vi "Vision_Processing_R_R5.vi"(0 "Current State":T6(ring)=enum."Short Range", 1 "Image Dst":T5=refnum, 2 "Inpute Image":T5=refnum, 3 "Startup Flag":bool, 5 "Current ROI Descriptor":T11={"Global Rectangle"=[0, 0, 320, 240], "Contours"=[{"ID"=enum."External", "Type"=12, "Coordinates"=[0, 0, 320, 240, 0]}]} {"Contours"."Type" items=["No Selection", "Point", "Line", "Rectangle", "Oval", "Polygon", "Freehand Region", "Annulus", "Unused2", "Unused3", "Broken Line", "Freehand Line", "Rotated Rectangle"]}, 6 "Avg Score - Last":dbl=802.5034383138021, 7 "error in (no error)":errorcluster, 8 "Current Settings":T9={"Curve Parameters"={"Extraction Mode"=1, "Edge Threshold"=150, "Edge Filter Size"=0, "Min Length"=25, "Row Search Step Size"=15, "Col Search Step Size"=15, "Max Endpoint Gap"=2, "Closed"=TRUE, "Subpixel"=TRUE}, "Match Mode"={"Rotation"=TRUE, "Scale"=TRUE, "Occlusion"=TRUE, "Reserved"=FALSE, "Reserved"=FALSE, "Reserved"=FALSE}, "Range Settings"=[{"Match Constraints"=0, "Min"=-5.0, "Max"=5.0}, {"Match Constraints"=1, "Min"=20.0, "Max"=150.0}, {"Match Constraints"=2, "Min"=0.0, "Max"=25.0}], "Number of Matches"=1, "Minimum Match Score"=800.0, "SubPixel Accuracy"=TRUE, "Adv. Geometric Match Options 2"=[{"Setup Data Item"=20, "Item Value"=0.0}, {"Setup Data Item"=22, "Item Value"=1.0}]} {"Curve Parameters"."Extraction Mode" items=["Normal", "Uniform Regions"]; "Curve Parameters"."Edge Filter Size" items=["Fine", "Normal", "Contour Tracing"]; "Curve Parameters"."Max Endpoint Gap" min=0; "Curve Parameters"."Col Search Step Size" min=1 max=255 step=1; "Curve Parameters"."Row Search Step Size" min=1 max=255 step=1; "Curve Parameters"."Min Length" min=0; "Curve Parameters"."Edge Threshold" min=1 max=350 step=1; "Range Settings"."Max" format="%.2f"; "Range Settings"."Min" format="%.2f"; "Range Settings"."Match Constraints" items=["Rotation Angle (degrees)", "Scale Factor (%)", "Occlusion (%)"]; "Adv. Geometric Match Options 2"."Setup Data Item" items=["Curve Extraction Mode", "Curve Edge Threshold", "Curve Edge Filter Size", "Min Curve Length", "Curve Row Search Step Size", "Curve Col Search Step Size", "Curve Max Endpoint Gap", "Extract Closed Curves", "Enable Subpixel Curve Extraction", "Enable Correlation Score", "Enable Subpixel Accuracy", "Subpixel Iterations", "Subpixel Tolerance", "Initial Match List Length", "Enable Target Template Curve Score", "Min Match Separation Distance", "Min Match Separation Angle", "Min Match Separation Scale", "Max Match Overlap", "Enable Coarse Result", "Enable Calibration Support", "Enable Contrast Reversal", "Search Strategy", "Refinement Match Factor", "Subpixel Match Factor"]}, 9 "Sub Beacon Search Enable":bool[](array[boolean])=[FALSE, FALSE, FALSE, FALSE, FALSE], 10 "History Data - IN":T4={"Valid Beacon History - in"=[FALSE, FALSE, FALSE, FALSE, FALSE, FALSE, FALSE, FALSE, FALSE, FALSE, FALSE, FALSE, FALSE, FALSE, FALSE, FALSE, FALSE, FALSE, FALSE, FALSE], "Valid Score History"=[916.1194458007812, 0.0, 921.171142578125, 952.2998657226562, 947.6416015625, 946.7607421875, 946.6710815429688, 913.2891235351562, 946.3783569335938, 946.1008911132812, 949.7362060546875, 948.7965087890625, 947.1905517578125, 948.5363159179688, 949.03466796875, 951.10986328125, 800.9814453125, 952.3334350585938, 926.0540161132812, 946.85888671875], "Valid Scale History"=[77.35153198242188, 0.0, 77.18988037109375, 76.20046997070312, 76.42532348632812, 76.47498321533203, 76.45317840576172, 77.11006927490234, 76.4490966796875, 76.39661407470703, 76.34481048583984, 76.36200714111328, 76.56851196289062, 76.3750228881836, 76.43797302246094, 76.20098876953125, 68.23258972167969, 76.18832397460938, 77.75858306884766, 76.44164276123047]} {"Valid Scale History" format="%#_13g"; "Valid Score History" format="%#_13g"}, 13 "Avg Scale - Last":dbl=73.9835688273112, 16 "History Size":i32=20) -> (11 "Avg Scale":dbl=73.9835688273112, 12 "Avg Score":dbl=802.5034383138021, 14 "Tracking Info":T1, 15 "Next Main ROI Descriptor":T2 {"Contours"."Type" items=["No Selection", "Point", "Line", "Rectangle", "Oval", "Polygon", "Freehand Region", "Annulus", "Unused2", "Unused3", "Broken Line", "Freehand Line", "Rotated Rectangle"]}, 17 "Beacon - Scales":sgl[](array[numeric])=[0.0, 0.0, 133.74268, 128.61499, 0.0], 18 "History Data - Out":T3={"Valid Beacon History\nOut"=[FALSE, FALSE, FALSE, FALSE, FALSE, FALSE, FALSE, FALSE, FALSE, FALSE, FALSE, FALSE, FALSE, FALSE, FALSE, FALSE, FALSE, FALSE, FALSE, FALSE], "Valid Score History\nOut"=[916.1194458007812, 0.0, 921.171142578125, 952.2998657226562, 947.6416015625, 946.7607421875, 946.6710815429688, 913.2891235351562, 946.3783569335938, 946.1008911132812, 949.7362060546875, 948.7965087890625, 947.1905517578125, 948.5363159179688, 949.03466796875, 951.10986328125, 800.9814453125, 952.3334350585938, 926.0540161132812, 946.85888671875], "Valid Scale History\nOut"=[77.35153198242188, 0.0, 77.18988037109375, 76.20046997070312, 76.42532348632812, 76.47498321533203, 76.45317840576172, 77.11006927490234, 76.4490966796875, 76.39661407470703, 76.34481048583984, 76.36200714111328, 76.56851196289062, 76.3750228881836, 76.43797302246094, 76.20098876953125, 68.23258972167969, 76.18832397460938, 77.75858306884766, 76.44164276123047]} {"Valid Scale History\nOut" format="%#_13g"; "Valid Score History\nOut" format="%#_13g"}, 19 "Y Coordinates":sgl[](array[numeric])=[0.0, 0.0, 133.74268, 128.61499, 0.0], 20 "Beacons Found":bool[](array[boolean])=[FALSE, FALSE, TRUE, TRUE, FALSE], 21 "X Coordinates":sgl[](array[numeric])=[0.0, 0.0, 162.26208, 213.98871, 0.0], 23 "Lock Status":bool, 24 "Startup Flag - out":bool, 25 "New Settings":T9={"Curve Parameters"={"Extraction Mode"=1, "Edge Threshold"=150, "Edge Filter Size"=0, "Min Length"=25, "Row Search Step Size"=15, "Col Search Step Size"=15, "Max Endpoint Gap"=2, "Closed"=TRUE, "Subpixel"=TRUE}, "Match Mode"={"Rotation"=TRUE, "Scale"=TRUE, "Occlusion"=TRUE, "Reserved"=FALSE, "Reserved"=FALSE, "Reserved"=FALSE}, "Range Settings"=[{"Match Constraints"=0, "Min"=-5.0, "Max"=5.0}, {"Match Constraints"=1, "Min"=20.0, "Max"=150.0}, {"Match Constraints"=2, "Min"=0.0, "Max"=25.0}], "Number of Matches"=1, "Minimum Match Score"=800.0, "SubPixel Accuracy"=TRUE, "Adv. Geometric Match Options 2"=[{"Setup Data Item"=20, "Item Value"=0.0}, {"Setup Data Item"=22, "Item Value"=1.0}]} {"Curve Parameters"."Extraction Mode" items=["Normal", "Uniform Regions"]; "Curve Parameters"."Edge Filter Size" items=["Fine", "Normal", "Contour Tracing"]; "Curve Parameters"."Max Endpoint Gap" min=0; "Curve Parameters"."Col Search Step Size" min=1 max=255 step=1; "Curve Parameters"."Row Search Step Size" min=1 max=255 step=1; "Curve Parameters"."Min Length" min=0; "Curve Parameters"."Edge Threshold" min=1 max=350 step=1; "Range Settings"."Max" format="%.2f"; "Range Settings"."Min" format="%.2f"; "Range Settings"."Match Constraints" items=["Rotation Angle (degrees)", "Scale Factor (%)", "Occlusion (%)"]}, 26 "Next State":T6(ring)=enum."Short Range", 27 "Right Image 2":T5(plugin-control))   [LabVIEW 2015]
uses:
  <vilib>/vision/Image Controls.llb/IMAQ Image.ctl
  <vilib>/vision/Pattern Matching.llb/IMAQ Curve Parameters.ctl
  <vilib>/vision/Pattern Matching.llb/IMAQ Match Range Setting.ctl
panel:
  in  "dimension size":i32=40
  in  "Divider (Filters 1)":sgl=1.0
  in  "SR / SCR\nTransition Scale":sgl=100.0
  in  "Score\nCushion- tight":dbl=75.0
  in  "Main ROI Decay\nper Fail (Vertical)":i32=5
  in  "ROI_factor(Horiztonal) SCR":sgl=1.7
  in  "ROI_factor(vertical) SCR":sgl=1.5
  in  "Dumping Range Beacon Filepath**":path=path "/home/lvuser/natinst/bin/BeaconTemplates/SCR_RIGHT.png"
  in  "Scale Decay \nFactor":dbl=0.5
  in  "Scale Decay \nFactor":dbl=5.0
  in  "Valid Treshold\nfor Lock":i16=3
  in  "Horiztonall Beacon \nCushion (pixels)":sgl=25.0
  out "New Min Score":dbl=800.0
  out "New Low Scale":dbl=20.0
  out "New high Scale":dbl=150.0
  in  "Absolute\nMinimum Score":dbl=700.0
  in  "Absolute\nMaximum Scale":dbl=300.0
  in  "Absolute\nMinimum Scale":dbl=10.0
  in  "Default No Lock\nSetting Values":T10={"Min Scale"=20.0, "Max Scale"=170.0, "Min Score"=800.0}
  in  "Score\nCushion":dbl=125.0
  in  "Scale \nCushion":dbl=7.0
  in  "LR to SR\nTransition Scale":sgl=80.0
  in  "SR /  LR\nTransition Scale":sgl=80.0
  in  "Timeout \nThrehsold":i32=1000
  in  "Main ROI Decay\nper Fail (Horiztonal)":i32=25
  in  "ROI_factor(Horiztonal) LR":sgl=5.0
  in  "ROI_factor(vertical) LR":sgl=1.5
  in  "ROI_factor(vertical) SR":sgl=2.7
  in  "ROI_factor(Horiztonal) SR":sgl=2.0
  out "Current  Score":sgl=916.11945
  out "Current  Scale":sgl=77.35153
  in  "Fail Count - In":i32
  in  "Sub Beacon Template File Path - ARRAY":path[](array[path])=[path "/home/lvuser/natinst/bin/BeaconTemplates/Sub1.png", path "/home/lvuser/natinst/bin/BeaconTemplates/Sub2.png", path "/home/lvuser/natinst/bin/BeaconTemplates/Sub3.png", path "/home/lvuser/natinst/bin/BeaconTemplates/Sub4.png", path "/home/lvuser/natinst/bin/BeaconTemplates/Sub5.png"]
  in  "Short Range Template FIle Path":path=path "/home/lvuser/natinst/bin/BeaconTemplates/SR_Right.png"
  in  "Long Range Main\nBeacon File Path":path=path "/home/lvuser/natinst/bin/BeaconTemplates/LR_Main.png"
  # "INPUTS"
  # "FILE PATHS"
  # "CONFIG"
  # "OUTPUTS"
  # "************"
  # "Range"
  # "Range"
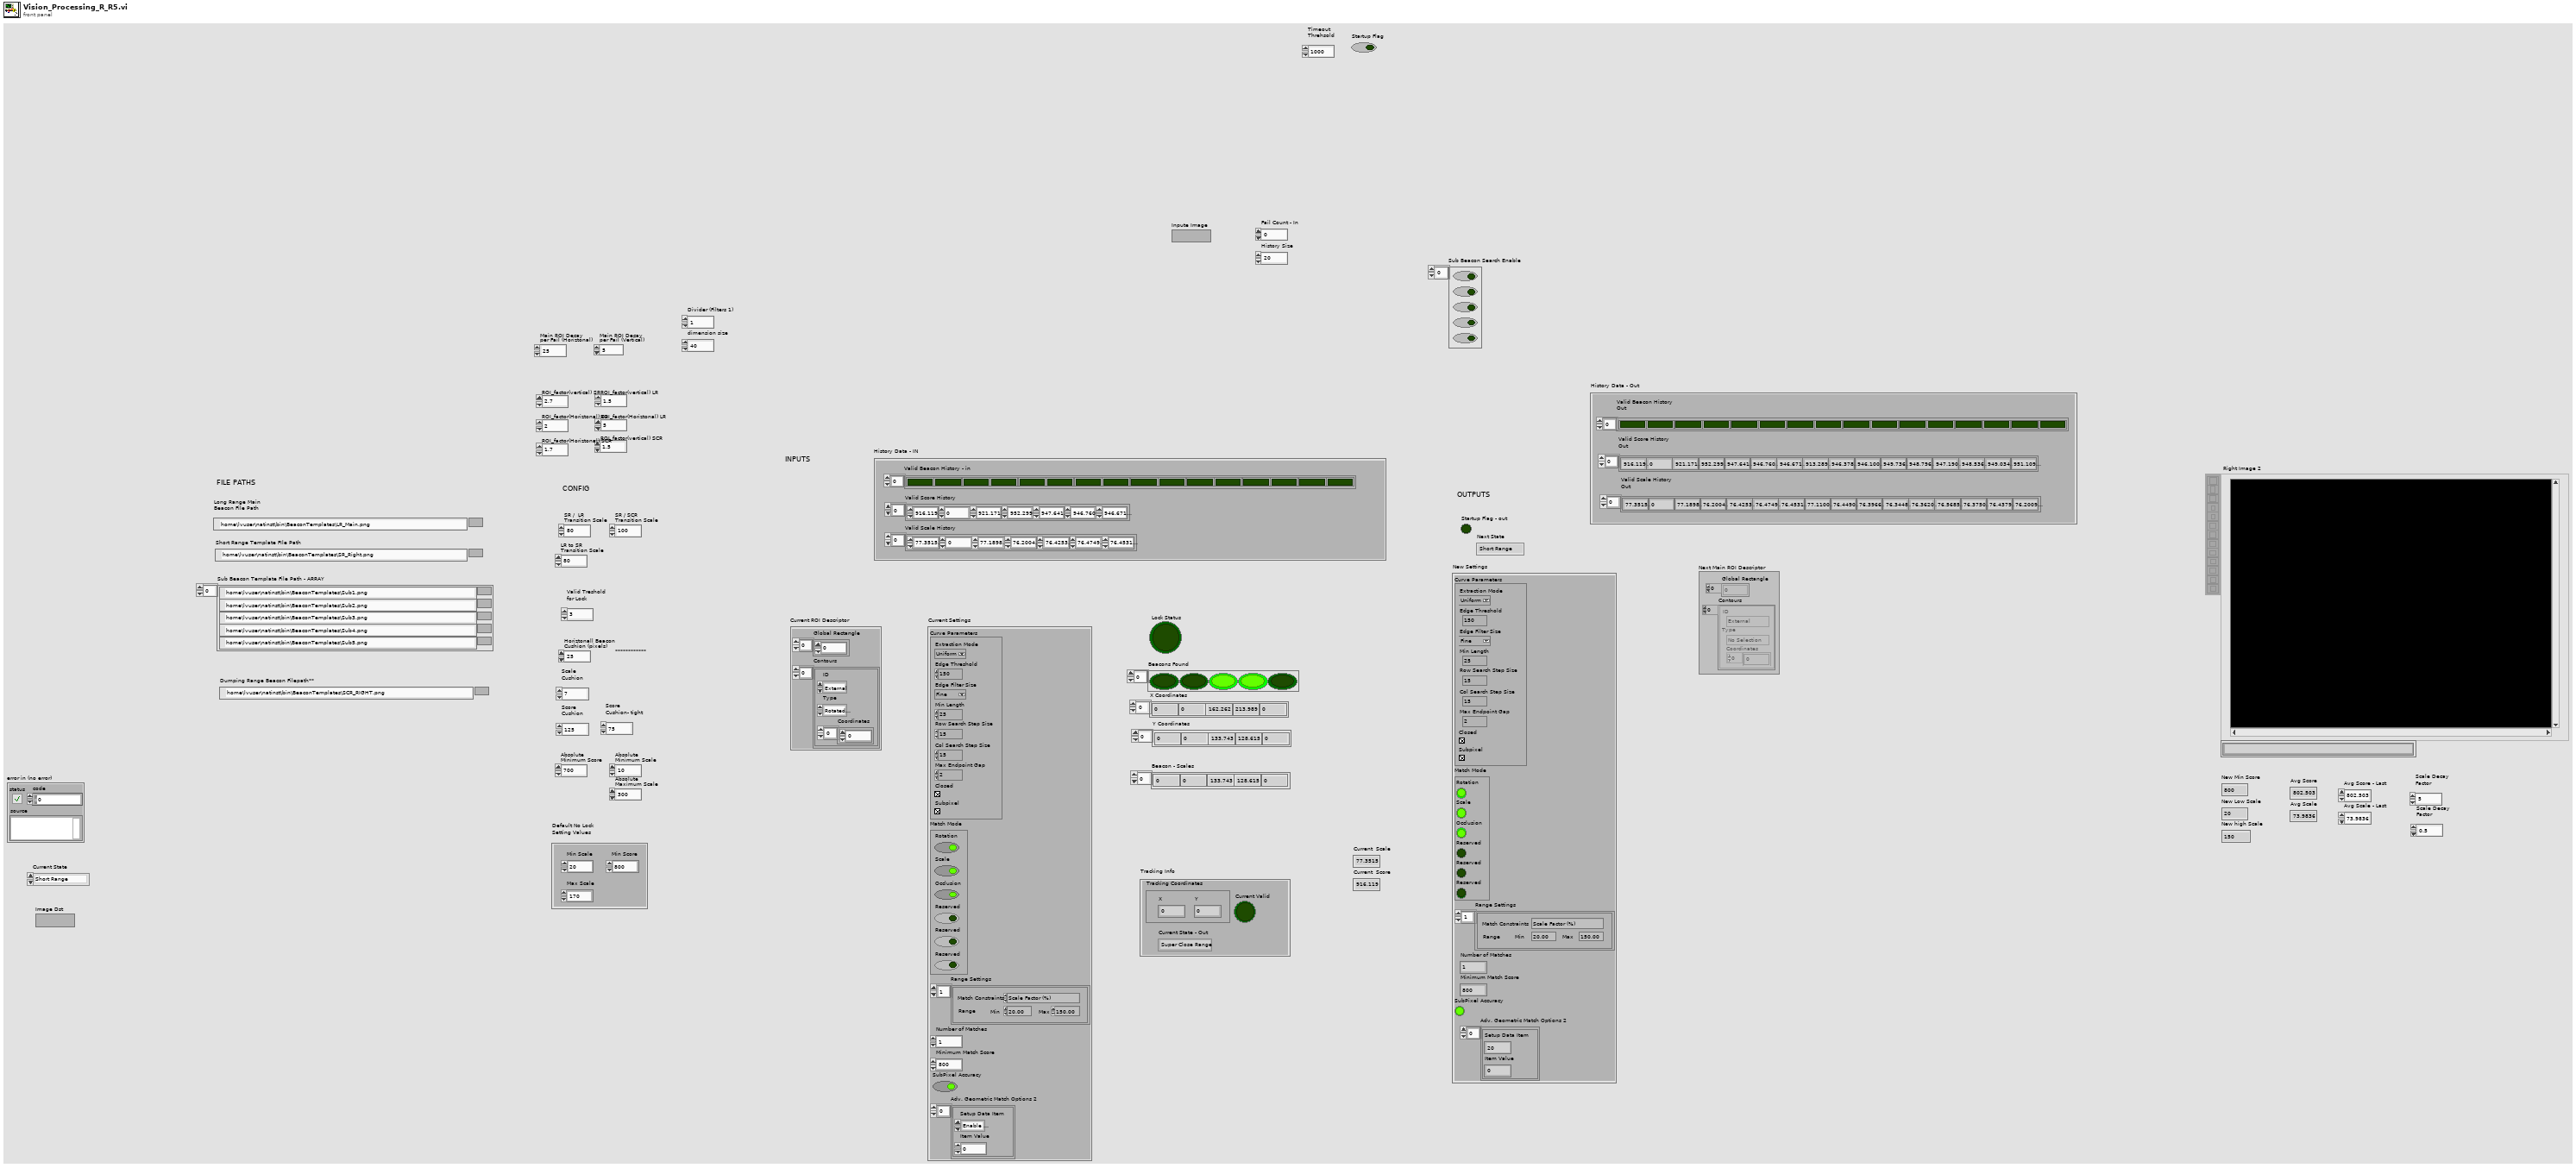
[diagram p1: front panel]
types:
  T1 = cluster{"Tracking Coordinates":cluster{"X":dbl, "Y":dbl}, "Current Valid":bool, "Current State - Out":enum16{"Super Close Range", "Short Range", "Long Range"}}
  T2 = typedef "ROI Descriptor" = cluster{"Global Rectangle":i32[], "Contours":cluster{"ID":enum32{"External", "Internal"}, "Type":u32, "Coordinates":i32[]}[]}
  T3 = cluster{"Valid Beacon History\nOut":bool[], "Valid Score History\nOut":dbl[], "Valid Scale History\nOut":dbl[]}
  T4 = cluster{"Valid Beacon History - in":bool[], "Valid Score History":dbl[], "Valid Scale History":dbl[]}
  T5 = typedef "IMAQ Image.ctl" = refnum<image>
  T6 = enum16{"Super Close Range", "Short Range", "Long Range"}
  T7 = typedef "IMAQ Curve Parameters.ctl" = cluster{"Extraction Mode":u32, "Edge Threshold":i32, "Edge Filter Size":u32, "Min Length":i32, "Row Search Step Size":i32, "Col Search Step Size":i32, "Max Endpoint Gap":i32, "Closed":bool, "Subpixel":bool}
  T8 = typedef "IMAQ Match Range Setting.ctl" = cluster{"Match Constraints":u32, "Min":dbl, "Max":dbl}
  T9 = cluster{"Curve Parameters":T7, "Match Mode":cluster{"Rotation":bool, "Scale":bool, "Occlusion":bool, "Reserved":bool, "Reserved":bool, "Reserved":bool}, "Range Settings":T8[], "Number of Matches":i32, "Minimum Match Score":sgl, "SubPixel Accuracy":bool, "Adv. Geometric Match Options 2":cluster{"Setup Data Item":u16, "Item Value":dbl}[]}
  T10 = cluster{"Min Scale":dbl, "Max Scale":dbl, "Min Score":dbl}
  T11 = cluster{"Global Rectangle":i32[], "Contours":cluster{"ID":enum32{"External", "Internal"}, "Type":u32, "Coordinates":i32[]}[]}
  T12 = typedef "IMAQ GM Match Report.ctl" = cluster{"Position":cluster{"x":sgl, "y":sgl}, "Angle":sgl, "Scale":sgl, "Score":sgl, "Bounding Box":cluster{"x":sgl, "y":sgl}[], "Contrast Reversed":bool, "Occlusion %":sgl, "Template Target Curve Score":sgl, "Target Template Curve Score":sgl, "Correlation Score":sgl}
  T13 = cluster{"Matches (Geometric Matching 1)[0]":T12, "Matches (Geometric Matching 1)[1]":T12, "Matches (Geometric Matching 1)[2]":T12, "Matches (Geometric Matching 1)[3]":T12, "Matches (Geometric Matching 1)[4]":T12, "Matches (Geometric Matching 1)[5]":T12, "Matches (Geometric Matching 1)[6]":T12, "Matches (Geometric Matching 1)[7]":T12, "Matches (Geometric Matching 1)[8]":T12}
  T14 = cluster{"Bounding Box[0]":cluster{"x":sgl, "y":sgl}, "Bounding Box[1]":cluster{"x":sgl, "y":sgl}, "Bounding Box[2]":cluster{"x":sgl, "y":sgl}, "Bounding Box[3]":cluster{"x":sgl, "y":sgl}, "Bounding Box[4]":cluster{"x":sgl, "y":sgl}, "Bounding Box[5]":cluster{"x":sgl, "y":sgl}, "Bounding Box[6]":cluster{"x":sgl, "y":sgl}, "Bounding Box[7]":cluster{"x":sgl, "y":sgl}, "Bounding Box[8]":cluster{"x":sgl, "y":sgl}}
  T15 = cluster{"Position":cluster{"x":sgl, "y":sgl}, bool, "Current State":enum16{"Super Close Range", "Short Range", "Long Range"}}
  T16 = typedef "IMAQ Rectangle" = cluster{"Left":i32, "Top":i32, "Right":i32, "Bottom":i32, "Rotation":dbl}
  T17 = cluster{"index":u32, "Min Scale":dbl, "Max Scale":dbl}
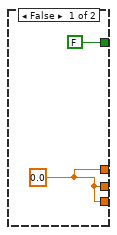
[diagram p2: hidden frame]
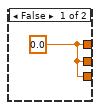
[diagram p3: hidden frame]
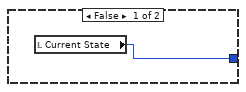
[diagram p7: hidden frame]
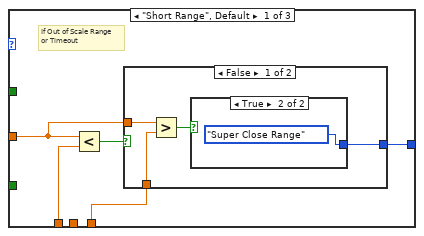
[diagram p8: hidden frame]
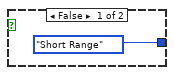
[diagram p9: hidden frame]
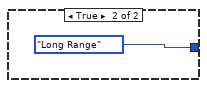
[diagram p10: hidden frame]
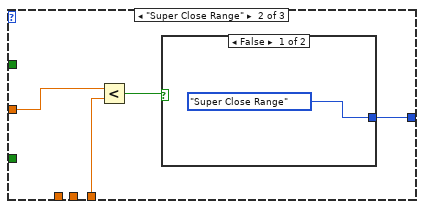
[diagram p11: hidden frame]
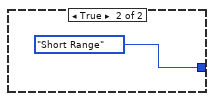
[diagram p12: hidden frame]
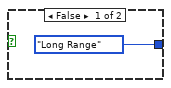
[diagram p13: hidden frame]
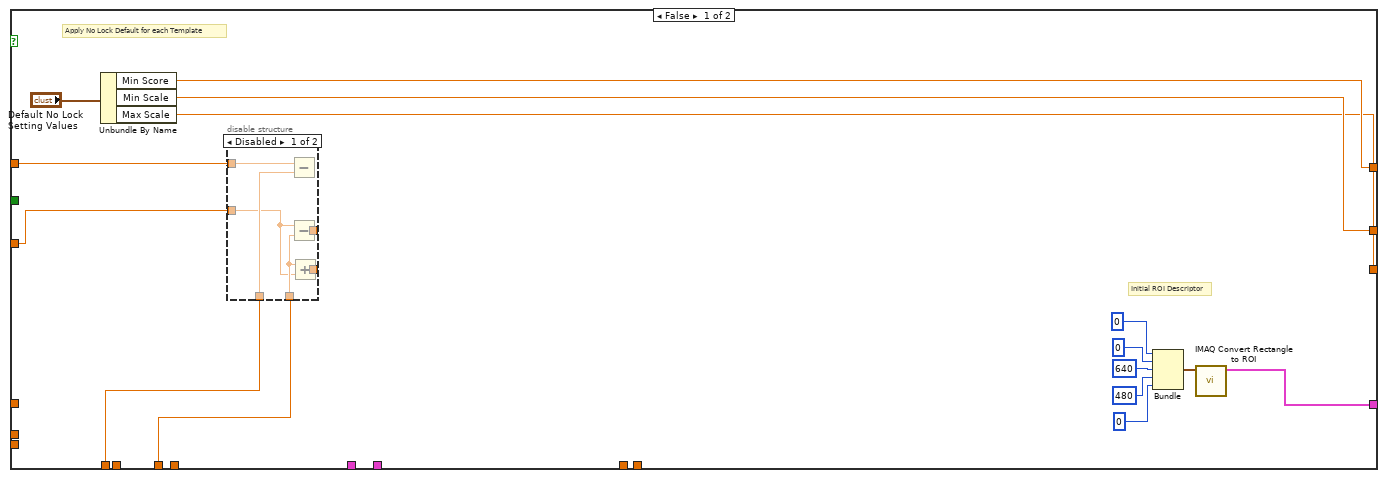
[diagram p15: hidden frame]
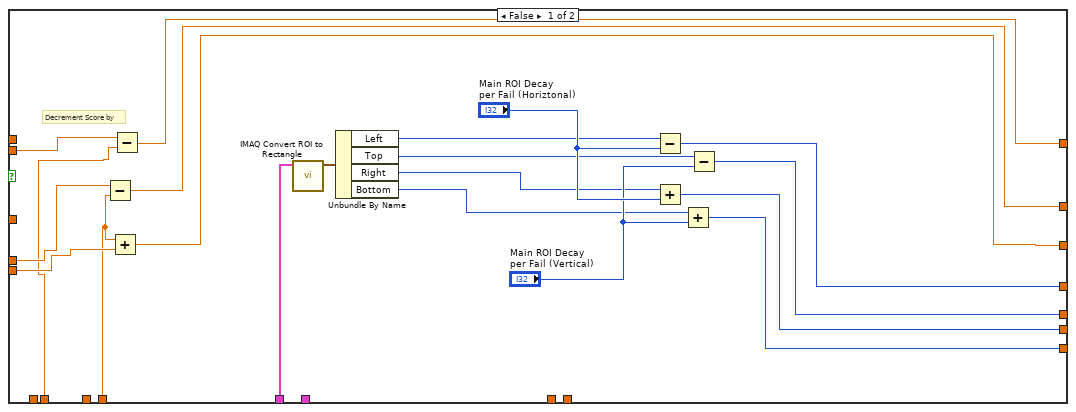
[diagram p17: hidden frame]
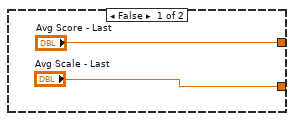
[diagram p18: hidden frame]
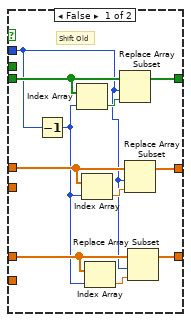
[diagram p20: hidden frame]
diagram:
  (unwired) enum16{"Short Range", "Long Range"}."Short Range"
  # "Next Settings"
  n1 = Initialize Array(sgl -1.0 ("element"), "dimension size", "dimension size") -> ()  [unwired: 1 out]
  n2 = flat-sequence {
    tunnel: [w10] -> w5
    tunnel: [w9] -> w4
    tunnel: ["Image Dst"] -> w3
    tunnel: w5 -> [w133]
    tunnel: w4 -> [w131]
    tunnel: w3 -> [w132]
    frame #0 {
      # "APPLY FILTERING"
      n3 = call "Camera - Filtering"("Image In"="Inpute Image", "Image Dst"="Image Dst", "error in"="error in (no error)") -> ("Image Out"=w10:T5, "error out"=w9:errorcluster)  [unwired: 23 in]
    }
    frame #1 {
      w92 = u32 1 ("index")
      w113 = u8 5
      # "Current is Valid"
      # "Update Tracking Coordinates"
      # "CURRENT VALID"
      # "*************"
      # "Beacon - Y"
      # "Beacon - X"
      # "Beacons Found"
      # "Build ROI for Individual Beacons Based on Main Bounding Box"
      # "Starting X Lower Bound"
      # "Length of\nIndividual Beacon ROI"
      # "Length of Bounding Box"
      # "Force SCR if Flagged"
      # "Choose ROI Factor based on Next State"
      # "Current Match"
      # "Current ROI"
      # "Image Lock"
      # "Force SR on Startup"
      # "Valid History"
      # "Draw ROI and stuff on outputi mage"
      # "Pull Down Startup IF Already True and Lock\nOtherwise don't update"
      # "Next Settings"
      # "Apply Limits to Settings"
      # "Scale"
      # "Min Score"
      # "Lower Scale"
      # "Upper Scale"
      # "Current Settings"
      # "Current Min\n& Max Scale"
      # "Current Valid"
      # "Update Search Settings"
      # "Update Template State"
      # "Calculate Average Scale/Score"
      # "max avg"
      # "Min Required to use avarage"
      # "Valid  Ccount\n(up to 3)"
      # "****# of previous in history that must be true\nin order for position to be considered \"locked\""
      # "Update Shift Arrays"
      # "# of Beacons Found to be valid"
      # "# of beacons"
      # "Matches"
      # "image out"
      n4 = Select(t=T6."Short Range", s="Startup Flag", f="Current State") -> (s? t:f=w11:T6)
      n5 = case shown="\"Short Range\"" w11 {
        tunnel: w133 -> [w396 w430 w463]
        tunnel: w132 -> [w395 w429 w462]
        tunnel: "Current ROI Descriptor" -> [w393 w427 w461]
        tunnel: "Current Settings" -> [w392 w426 w460]
        tunnel: [w388 w422 w456] -> w49
        tunnel: [w389 w421 w455] -> w72
        tunnel: [w390 w419 w453] -> w122
        tunnel: w131 -> [w394 _ w452]
        tunnel: "Sub Beacon Search Enable" -> [w397 w420 w451]
        tunnel: [2.0 sgl 3.0 ("y") sgl 5.0 ("y")] -> w129
        tunnel: [w386 w417 w449] -> w128
        tunnel: [1 2 3] -> w123
        frame "Super Close Range", Default {
          # "**Make sure this selects the \nbeacon used for close range!!!"
          n6 = call "Dumping Range"("Image In"=w396, "Image Dst"=w395, "ROI Descriptor (Geometric Matching 1)"=w393, "Settings (Geometric Matching 1)"=w392, "Template File Path (Geometric Matching 1)"="Dumping Range Beacon Filepath**", "error in"=w394) -> ("Image Out"=w389:T5, "Matches (Geometric Matching 1)"=w388:T12[], "Number of Matches (Geometric Matching 1)"=w385:i32, "error out"=w386:errorcluster)  [unwired: 18 in]
          n7 = Equal?(x=w385, y=1) -> (x = y?=w383:bool)
          n8 = case shown="True" w383 {
            tunnel: w397 -> [w406 w409]
            tunnel: [w399 w410] -> w390
            frame False {
              w400 = FALSE
              # "F"
              # "No Main Found,\nDon't Search any Subs"
              n9 = Replace Array Subset(array=w406, new element #1=w400, index #1=0 ("y"), new element #2=w400, index #2=1 ("y"), new element #3=w400, index #3=2 ("y"), new element #4=w400, index #4=3 ("y"), new element #5=w400, index #5=4 ("y")) -> (w399:bool[])
            }
            frame True {
              w408 = TRUE
              w407 = FALSE
              # "Search for MIDDLE Beacons"
              n10 = Replace Array Subset(array=w409, new element #1=w407, index #1=0 ("y"), new element #2=w407, index #2=1 ("y"), new element #3=w407, index #3=2 ("y"), new element #4=w408, index #4=3 ("y"), new element #5=w408, index #5=4 ("y")) -> (w410:bool[])
            }
          }
        }
        frame "Short Range" {
          n11 = call "Short Range"("Image In"=w430, "Image Dst"=w429, "ROI Descriptor (Geometric Matching 1)"=w427, "Settings (Geometric Matching 1)"=w426, "Template File Path (Geometric Matching 1)"="Short Range Template FIle Path") -> ("Image Out"=w421:T5, "Matches (Geometric Matching 1)"=w422:T12[], "Number of Matches (Geometric Matching 1)"=w423:i32, "error out"=w417:errorcluster)  [unwired: 19 in]
          n12 = Equal?(x=w423, y=1) -> (x = y?=w424:bool)
          n13 = case shown="True" w424 {
            tunnel: w420 -> [w438 w441]
            tunnel: [w431 w442] -> w419
            frame False {
              w432 = FALSE
              # "F"
              # "No Main Found,\nDon't Search any Subs"
              n14 = Replace Array Subset(array=w438, new element #1=w432, index #1=0 ("y"), new element #2=w432, index #2=1 ("y"), new element #3=w432, index #3=2 ("y"), new element #4=w432, index #4=3 ("y"), new element #5=w432, index #5=4 ("y")) -> (w431:bool[])
            }
            frame True {
              w440 = TRUE
              w439 = FALSE
              # "Search for specific Beacons"
              n15 = Replace Array Subset(array=w441, new element #1=w439, index #1=0 ("y"), new element #2=w439, index #2=1 ("y"), new element #3=w440, index #3=2 ("y"), new element #4=w440, index #4=3 ("y"), new element #5=w440, index #5=4 ("y")) -> (w442:bool[])
            }
          }
        }
        frame "Long Range" {
          n16 = call "Long Range"("Image In"=w463, "Image Dst"=w462, "ROI Descriptor (Geometric Matching 1)"=w461, "Settings (Geometric Matching 1)"=w460, "Template File Path (Geometric Matching 1)"="Long Range Main\nBeacon File Path", "error in"=w452) -> ("Image Out"=w455:T5, "Matches (Geometric Matching 1)"=w456:T12[], "Number of Matches (Geometric Matching 1)"=w458:i32, "error out"=w449:errorcluster)  [unwired: 18 in]
          n17 = Equal?(x=w458, y=1) -> (x = y?=w454:bool)
          n18 = case shown="True" w454 {
            tunnel: w451 -> [w471 w473]
            tunnel: [w464 w472] -> w453
            frame False {
              w465 = FALSE
              # "F"
              # "No Main Found,\nDon't Search any Subs"
              n19 = Replace Array Subset(array=w471, new element #1=w465, index #1=0 ("y"), new element #2=w465, index #2=1 ("y"), new element #3=w465, index #3=2 ("y"), new element #4=w465, index #4=3 ("y"), new element #5=w465, index #5=4 ("y")) -> (w464:bool[])
            }
            frame True {
              w474 = TRUE
              # "T"
              # "Search for ALL Beacons"
              n20 = Replace Array Subset(array=w473, new element #1=w474, index #1=0 ("y"), new element #2=w474, index #2=1 ("y"), new element #3=w474, index #3=2 ("y"), new element #4=w474, index #4=3 ("y"), new element #5=w474, index #5=4 ("y")) -> (w472:bool[])
            }
          }
        }
      }
      n21 = Array To Cluster(array=w49) -> (cluster=w39:T13)
      n22 = Unbundle By Name(w39) -> ("Matches (Geometric Matching 1)[0].Position"=w13:cluster{"x":sgl, "y":sgl}, "Matches (Geometric Matching 1)[0].Bounding Box"=w37:cluster{"x":sgl, "y":sgl}[], "Matches (Geometric Matching 1)[0].Scale"=w71:sgl, "Matches (Geometric Matching 1)[0].Score"=w83:sgl)
      "Current  Scale" <- w71
      "Current  Score" <- w83
      n23 = Array To Cluster(array=w37) -> (cluster=w38:T14)
      n24 = Unbundle By Name(w38) -> ("Bounding Box[0].x"=w28:sgl, "Bounding Box[0].y"=w27:sgl, "Bounding Box[2].x"=w26:sgl, "Bounding Box[2].y"=w25:sgl)
      n25 = Bundle("x"=w28, "y"=w27, "x"=w26, "y"=w25) -> (w23:cluster{"x":sgl, "y":sgl, "x":sgl, "y":sgl})  [unwired: 1 in]
      n26 = call "IMAQ Overlay Rectangle"("Rectangle"=w23, "Image"=w72) -> ("Image Out"=w24:T5)  [unwired: 8 in, 1 out]
      n27 = Subtract(x=w26, y=w28) -> (x-y=w32:sgl)
      n28 = Divide(x=w32, y=w129) -> (x/y=w34:dbl)
      n29 = Multiply(x="Horiztonall Beacon \nCushion (pixels)", y=w71) -> (x*y=w22:sgl)
      n30 = Divide(x=w22, y=sgl 100.0) -> (x/y=w19:sgl)
      n31 = Subtract(x=w27, y=w19) -> (x-y=w35:sgl)
      n32 = Add(x=w19, y=w25) -> (x+y=w36:sgl)
      n33 = for {
        N: 5 -> [_]
        tunnel: w122 -> [w176] mode=indexing
        shift-right: [w170] -> _
        shift-left: w28 -> [w175]
        tunnel: w34 -> [w174]
        tunnel: w35 -> [w167]
        tunnel: w36 -> [w166]
        tunnel: [w173] -> w30 mode=indexing
        tunnel: w19 -> [w168]
        # "Divide Bounding Box"
        # "Upper Bound of Current is\nLower Bound for Next"
        n34 = case shown="True" w176 {
          tunnel: w175 -> [w177 w178]
          tunnel: w174 -> [_ w180]
          tunnel: [w177 w179] -> w170
          tunnel: [w177 w178] -> w172
          frame False {
            # "Don't Care"
          }
          frame True {
            # "X Lower Bound"
            n35 = Add(x=w178, y=w180) -> (x+y=w179:dbl)
          }
        }
        n36 = Subtract(x=w172, y=w168) -> (x-y=w171:dbl)
        n37 = Add(x=w170, y=w168) -> (x+y=w169:dbl)
        n38 = call "Bound_RO_R_R0I.vi"("Bottom Right - Y"=w166, "Right - X"=w169, "Top Left - Y"=w167, "Top  Left - x"=w171) -> ("ROI Descriptor"=w173:T2)  [unwired: 7 in]
      }
      n39 = for {
        N: 5 -> [_]
        tunnel: w72 -> [w145]
        tunnel: w128 -> [w144]
        tunnel: w30 -> [w137] mode=indexing
        tunnel: "Sub Beacon Template File Path - ARRAY" -> [w143] mode=indexing
        tunnel: [w142] -> w127 mode=indexing
        tunnel: [w141] -> w126 mode=indexing
        tunnel: [w140] -> w114 mode=indexing
        tunnel: w122 -> [w139] mode=indexing
        tunnel: "Current Settings" -> [w138]
        shift-right: [w135] -> w73
        shift-left: w24 -> [w136]
        tunnel: [w134] -> w62 mode=indexing
        n40 = case shown="True" w139 {
          tunnel: w145 -> [_ w159]
          tunnel: w144 -> [_ w158]
          tunnel: w137 -> [_ w157]
          tunnel: w143 -> [_ w156]
          tunnel: [w146 w152] -> w142
          tunnel: [w146 w151] -> w141
          tunnel: [FALSE w150] -> w140
          tunnel: w138 -> [_ w149]
          tunnel: [w146 w148] -> w134
          frame False {
            w146 = sgl 0.0 ("x")
          }
          frame True {
            n41 = call "Sub Beacon Pattern Match"("Image In"=w159, "ROI Descriptor (Geometric Matching 1)"=w157, "Settings (Geometric Matching 1)"=w149, "Template File Path (Geometric Matching 1)"=w156, "error in"=w158) -> ("Matches (Geometric Matching 1)"=w153:T12[], "Number of Matches (Geometric Matching 1)"=w154:i32)  [unwired: 19 in, 2 out]
            n42 = Equal?(x=w154, y=1) -> (x = y?=w150:bool)
            n43 = case shown="True" w150 {
              tunnel: w153 -> [_ w164]
              tunnel: [w160 w163] -> w152
              tunnel: [w160 w162] -> w151
              tunnel: [w160 w161] -> w148
              frame False {
                w160 = sgl 0.0 ("x")
              }
              frame True {
                n44 = Array To Cluster(array=w164) -> (cluster=w165:T13)
                n45 = Unbundle By Name(w165) -> ("Matches (Geometric Matching 1)[0].Position.x"=w163:sgl, "Matches (Geometric Matching 1)[0].Position.y"=w162:sgl, "Matches (Geometric Matching 1)[0].Scale"=w161:sgl)
              }
            }
          }
        }
        n46 = call "IMAQ Overlay ROI"("ROI Descriptor"=w137, "Image"=w136) -> ("Image Out"=w135:T5)  [unwired: 8 in, 1 out]
      }
      "Beacons Found" <- w114
      "X Coordinates" <- w127
      "Y Coordinates" <- w126
      "Beacon - Scales" <- w62
      n47 = Boolean To (0,1)(Boolean=w114) -> (0, 1=w124:i16[])
      n48 = Add Array Elements(numeric array=w124) -> (sum=w125:i16)
      n49 = Greater Or Equal?(x=w125, y=w123) -> (x >= y?=w12:bool)
      n50 = case shown="False" w12 {
        tunnel: "Fail Count - In" -> [w381 _]
        tunnel: [w380 u16 0] -> w106
        frame False {
          n51 = Increment(x=w381) -> (x+1=w380:i32)
        }
        frame True {
          # "reset fail count"
        }
      }
      n52 = Unbundle By Name("History Data - IN") -> ("Valid Beacon History - in"=w69:bool[], "Valid Score History"=w68:dbl[], "Valid Scale History"=w67:dbl[])
      n53 = Greater?(x=w106, y="Timeout \nThrehsold") -> (0:w15:bool)
      n54 = Decrement(x="History Size") -> (x-1=w120:i32)
      n55 = for {
        N: "History Size" -> [_]
        shift-right: [w358] -> w66
        shift-left: w69 -> [w346]
        tunnel: w120 -> [w354]
        shift-right: [w351] -> w65
        shift-left: w68 -> [w353]
        shift-right: [w350] -> w64
        shift-left: w67 -> [w352]
        tunnel: w83 -> [w349]
        tunnel: w71 -> [w348]
        tunnel: w12 -> [w347]
        i -> [w357]
        # "Reverse Index"
        n56 = Subtract(x=w354, y=w357) -> (x-y=w355:i32)
        n57 = Equal To 0?(x=w355) -> (x = 0?=w356:bool)
        n58 = case shown="True" w356 {
          tunnel: w355 -> [w359 w378]
          tunnel: w346 -> [w369 w371]
          tunnel: [w367 w370] -> w358
          tunnel: w347 -> [_ w379]
          tunnel: w353 -> [w364 w377]
          tunnel: w352 -> [w363 w376]
          tunnel: [w362 w374] -> w351
          tunnel: [w361 w375] -> w350
          tunnel: w349 -> [_ w373]
          tunnel: w348 -> [_ w372]
          frame False {
            # "Shift Old"
            n59 = Decrement(x=w359) -> (x-1=w360:i32)
            n60 = Index Array(array=w369, index=w360) -> (element=w368:bool)
            n61 = Index Array(array=w364, index=w360) -> (element=w366:dbl)
            n62 = Index Array(array=w363, index=w360) -> (element=w365:dbl)
            n63 = Replace Array Subset(array=w369, new element=w368, index=w359) -> (w367:bool[])
            n64 = Replace Array Subset(array=w364, new element=w366, index=w359) -> (w362:dbl[])
            n65 = Replace Array Subset(array=w363, new element=w365, index=w359) -> (w361:dbl[])
          }
          frame True {
            # "Scale"
            # "Score"
            # "Valid"
            # "insert New"
            n66 = Replace Array Subset(array=w377, new element=w373, index=w378) -> (w374:dbl[])
            n67 = Replace Array Subset(array=w376, new element=w372, index=w378) -> (w375:dbl[])
            n68 = Replace Array Subset(array=w371, new element=w379, index=w378) -> (w370:bool[])
          }
        }
      }
      n69 = Boolean To (0,1)(Boolean=w66) -> (0, 1=w118:i16[])
      n70 = Bundle("Valid Beacon History - in"=w66, "Valid Score History"=w65, "Valid Scale History"=w64) -> (→"History Data - Out":T4)  [unwired: 1 in]
      n71 = Add Array Elements(numeric array=w118) -> (sum=w119:i16)
      n72 = Greater Or Equal?(x=w119, y="Valid Treshold\nfor Lock") -> (x >= y?=w84:bool)
      "Lock Status" <- w84
      n73 = Initialize Array(u8 0, w113) -> (w116:u8[])
      n74 = while {
        shift-right: [w329] -> w111
        shift-left: w116 -> [w331]
        tunnel: w66 -> [w337] mode=indexing
        shift-right: [w335] -> w109
        shift-left: u8 0 -> [w338]
        tunnel: "History Size" -> [w336]
        tunnel: w113 -> [w328]
        i -> [w330]
        stop <- w332 stop-if-true
        # "Grab Last 2 Valid Indexes"
        n75 = case shown="True" w337 {
          tunnel: w338 -> [w340 w342]
          tunnel: [w340 w345] -> w335
          tunnel: w331 -> [w339 w344]
          tunnel: w330 -> [_ w343]
          tunnel: [w339 w341] -> w329
          frame False {
          }
          frame True {
            # "Update Index\nto use"
            # "Increment\nValid Count"
            n76 = Replace Array Subset(array=w344, new element=w343, index=w342) -> (w341:u8[])
            n77 = Increment(x=w342) -> (x+1=w345:u8)
          }
        }
        n78 = Greater?(x=w330, y=w336) -> (0:w333:bool)
        n79 = Greater Or Equal?(x=w335, y=w328) -> (x >= y?=w334:bool)
        n80 = Or(x=w334, y=w333) -> (x .or. y?=w332:bool)
      }
      n81 = Greater?(x=w109, y=u8 2) -> (0:w110:bool)
      n82 = case shown="True" w110 {
        tunnel: w109 -> [_ w312]
        tunnel: w111 -> [_ w318]
        tunnel: w65 -> [_ w317]
        tunnel: w64 -> [_ w316]
        tunnel: ["Avg Score - Last" w310] -> w80
        tunnel: ["Avg Scale - Last" w309] -> w81
        frame False {
        }
        frame True {
          w315 = 0.0
          n83 = for {
            N: w312 -> [_]
            tunnel: w318 -> [w325] mode=indexing
            tunnel: w317 -> [w327]
            tunnel: w316 -> [w326]
            shift-right: [w323] -> w314
            shift-left: w315 -> [w321]
            shift-right: [w324] -> w313
            shift-left: w315 -> [w320]
            # "Fetch Last Valid Values"
            n84 = Index Array(array=w327, index=w325) -> (element=w322:dbl)
            n85 = Index Array(array=w326, index=w325) -> (element=w319:dbl)
            n86 = Add(x=w322, y=w321) -> (x+y=w323:dbl)
            n87 = Add(x=w319, y=w320) -> (x+y=w324:dbl)
          }
          n88 = To Double Precision Float(number=w312) -> (double precision float=w311:dbl)
          n89 = Divide(x=w314, y=w311) -> (x/y=w310:dbl)
          n90 = Divide(x=w313, y=w311) -> (x/y=w309:dbl)
        }
      }
      "Avg Score" <- w80
      "Avg Scale" <- w81
      n91 = Bundle("Position"=w13, w12, "Current State"=w11) -> (→"Tracking Info":T15)  [unwired: 1 in]
      n92 = case shown="True" w84 {
        tunnel: w15 -> [_ w194]
        tunnel: "SR /  LR\nTransition Scale" -> [_ w193]
        tunnel: "LR to SR\nTransition Scale" -> [_ w192]
        tunnel: w81 -> [_ w191]
        tunnel: w84 -> [_ w190]
        tunnel: [w187 w189] -> w16
        tunnel: "SR / SCR\nTransition Scale" -> [_ w188]
        frame False {
          n93 = local read "Current State"() -> (w187:T6)
        }
        frame True {
          # "Timeout"
          # "Image Lock"
          n94 = local read "Current State"() -> (w195:T6)
          n95 = case shown="\"Long Range\"" w195 {
            tunnel: w190 -> [_ _ _]
            tunnel: w191 -> [w197 w210 w216]
            tunnel: w194 -> [_ _ _]
            tunnel: w193 -> [w200 _ _]
            tunnel: w192 -> [_ _ w215]
            tunnel: [w198 w208 w214] -> w189
            tunnel: w188 -> [w196 w211 _]
            frame "Short Range", Default {
              # "If Out of Scale Range\nor Timeout"
              n96 = Less?(x=w197, y=w200) -> (x < y?=w199:bool)
              n97 = case shown="False" w199 {
                tunnel: [w204 T6."Long Range"] -> w198
                tunnel: w197 -> [w202 _]
                tunnel: w196 -> [w201 _]
                frame False {
                  n98 = Greater?(x=w202, y=w201) -> (0:w203:bool)
                  n99 = case shown="True" w203 {
                    tunnel: [T6."Short Range" T6."Super Close Range"] -> w204
                    frame False {
                    }
                    frame True {
                    }
                  }
                }
                frame True {
                }
              }
            }
            frame "Super Close Range" {
              n100 = Less?(x=w210, y=w211) -> (x < y?=w209:bool)
              n101 = case shown="False" w209 {
                tunnel: [T6."Super Close Range" T6."Short Range"] -> w208
                frame False {
                }
                frame True {
                }
              }
            }
            frame "Long Range" {
              # "If Out of Scale Range\nor Timeout"
              n102 = Greater?(x=w216, y=w215) -> (0:w217:bool)
              n103 = case shown="True" w217 {
                tunnel: [T6."Long Range" T6."Short Range"] -> w214
                frame False {
                }
                frame True {
                }
              }
            }
          }
        }
      }
      "Next State" <- w16
      n104 = Unbundle By Name("Current Settings") -> ("Minimum Match Score"=w103:sgl, "Range Settings"=w89:T8[])
      n105 = case shown="\"Short Range\"" w16 {
        tunnel: "ROI_factor(vertical) SR" -> [_ _ w186]
        tunnel: "ROI_factor(Horiztonal) SR" -> [_ _ w185]
        tunnel: "ROI_factor(vertical) LR" -> [_ w184 _]
        tunnel: "ROI_factor(Horiztonal) LR" -> [_ w183 _]
        tunnel: "ROI_factor(vertical) SCR" -> [w182 _ _]
        tunnel: "ROI_factor(Horiztonal) SCR" -> [w181 _ _]
        tunnel: [w182 w184 w186] -> w42
        tunnel: [w181 w183 w185] -> w41
        frame "Super Close Range", Default {
        }
        frame "Long Range" {
        }
        frame "Short Range" {
        }
      }
      n106 = Index Array(array=w89, index=u32 1) -> (element=w102:T8)
      n107 = Unbundle(w102) -> ("Min"=w100:dbl, "Max"=w99:dbl)  [unwired: 1 out]
      n108 = case shown="True" w84 {
        tunnel: w12 -> [_ w264]
        tunnel: w80 -> [w233 w263]
        tunnel: w81 -> [w232 w262]
        tunnel: w103 -> [_ w261]
        tunnel: w100 -> [_ w260]
        tunnel: w99 -> [_ w259]
        tunnel: [w231 w250] -> w90
        tunnel: [w230 w249] -> w53
        tunnel: [w229 w248] -> w54
        tunnel: "Scale \nCushion" -> [w235 w258]
        tunnel: "Score\nCushion" -> [w234 w257]
        tunnel: "Scale Decay \nFactor" -> [_ w256]
        tunnel: "Scale Decay \nFactor" -> [_ w255]
        tunnel: "Current ROI Descriptor" -> [_ w251]
        tunnel: w49 -> [_ w252]
        tunnel: w42 -> [_ w254]
        tunnel: w41 -> [_ w253]
        tunnel: [w222 w247] -> w40
        frame False {
          # "Initial ROI Descriptor"
          # "Apply No Lock Default for each Template"
          n109 = Unbundle By Name("Default No Lock\nSetting Values") -> ("Min Score"=w231:dbl, "Min Scale"=w230:dbl, "Max Scale"=w229:dbl)
          n110 = disable-structure shown="Disabled" {
            disable-tunnel: [w242 _] -> _
            disable-tunnel: [w241 _] -> _
            disable-tunnel: w235 -> [w240 _]
            disable-tunnel: w234 -> [w239 _]
            disable-tunnel: w233 -> [w238 _]
            disable-tunnel: w232 -> [w237 _]
            frame Disabled {
              n111 = Subtract(x=w238, y=w239) -> ()  [unwired: 1 out]
              n112 = Subtract(x=w237, y=w240) -> (x-y=w242:dbl)
              n113 = Add(x=w240, y=w237) -> (x+y=w241:dbl)
            }
            frame Enabled {
            }
          }
          n114 = Bundle(0, 0, 640, 480, 0) -> (w228:cluster{i32, i32, i32, i32, i32})  [unwired: 1 in]
          n115 = call "IMAQ Convert Rectangle to ROI"("Rectangle"=w228) -> ("ROI Descriptor"=w222:T2)  [unwired: 8 in, 1 out]
        }
        frame True {
          # "Apply Limits to ROI"
          n116 = case shown="True" w264 {
            tunnel: w263 -> [_ w306]
            tunnel: [w279 w302] -> w250
            tunnel: w262 -> [_ w305]
            tunnel: [w278 w301] -> w249
            tunnel: [w277 w300] -> w248
            tunnel: w260 -> [w284 _]
            tunnel: w259 -> [w283 _]
            tunnel: w261 -> [w282 _]
            tunnel: w258 -> [_ w304]
            tunnel: w257 -> [_ w303]
            tunnel: w256 -> [w281 _]
            tunnel: w255 -> [w280 _]
            tunnel: w254 -> [_ w291]
            tunnel: w253 -> [_ w290]
            tunnel: w252 -> [_ w289]
            tunnel: [w268 w288] -> w246
            tunnel: [w267 w287] -> w245
            tunnel: [w266 w286] -> w244
            tunnel: [w265 w285] -> w243
            tunnel: w251 -> [w275 _]
            frame False {
              # "Decrement Score by"
              n117 = Subtract(x=w284, y=w280) -> (x-y=w278:dbl)
              n118 = Add(x=w280, y=w283) -> (x+y=w277:dbl)
              n119 = Subtract(x=w282, y=w281) -> (x-y=w279:dbl)
              n120 = call "IMAQ Convert ROI to Rectangle"("ROI Descriptor"=w275) -> ("Rectangle"=w276:T16)  [unwired: 8 in, 1 out]
              n121 = Unbundle By Name(w276) -> ("Left"=w272:i32, "Top"=w271:i32, "Right"=w270:i32, "Bottom"=w269:i32)
              n122 = Subtract(x=w272, y="Main ROI Decay\nper Fail (Horiztonal)") -> (x-y=w268:i32)
              n123 = Add(x=w270, y="Main ROI Decay\nper Fail (Horiztonal)") -> (x+y=w266:i32)
              n124 = Add(x=w269, y="Main ROI Decay\nper Fail (Vertical)") -> (x+y=w265:i32)
              n125 = Subtract(x=w271, y="Main ROI Decay\nper Fail (Vertical)") -> (x-y=w267:i32)
            }
            frame True {
              # "Scale / Score"
              # "Main ROI"
              # "Horizontal Scale \n(smaller number = smaller ROI)"
              n126 = Subtract(x=w306, y=w303) -> (x-y=w302:dbl)
              n127 = Subtract(x=w305, y=w304) -> (x-y=w301:dbl)
              n128 = Add(x=w304, y=w305) -> (x+y=w300:dbl)
              n129 = Array To Cluster(array=w289) -> (cluster=w299:T13)
              n130 = Unbundle By Name(w299) -> ("Matches (Geometric Matching 1)[0].Position.x"=w293:sgl, "Matches (Geometric Matching 1)[0].Position.y"=w295:sgl, "Matches (Geometric Matching 1)[0].Scale"=w294:sgl)
              n131 = Divide(x=w294, y=w291) -> (x/y=w296:sgl)
              n132 = Multiply(x=w294, y=w290) -> (x*y=w298:sgl)
              n133 = Divide(x=w298, y=sgl 2.0) -> (x/y=w292:sgl)
              n134 = Add(x=w295, y=w296) -> (x+y=w285:sgl)
              n135 = Subtract(x=w295, y=w296) -> (x-y=w287:sgl)
              n136 = Subtract(x=w293, y=w292) -> (x-y=w288:sgl)
              n137 = Add(x=w292, y=w293) -> (x+y=w286:sgl)
            }
          }
          n138 = call "Bound_RO_R_R0I.vi"("Bottom Right - Y"=w243, "Right - X"=w244, "Top Left - Y"=w245, "Top  Left - x"=w246) -> ("ROI Descriptor"=w247:T2)  [unwired: 7 in]
        }
      }
      "Next Main ROI Descriptor" <- w40
      n139 = And(x="Startup Flag", y=w84) -> (x .and. y?=w87:bool)
      n140 = case shown="True" w87 {
        tunnel: "Startup Flag" -> [w220 _]
        tunnel: [w220 FALSE] -> w86
        frame False {
        }
        frame True {
        }
      }
      "Startup Flag - out" <- w86
      n141 = Less?(x=w90, y="Absolute\nMinimum Score") -> (x < y?=w94:bool)
      n142 = Less?(x=w53, y="Absolute\nMinimum Scale") -> (x < y?=w56:bool)
      n143 = Greater?(x=w54, y="Absolute\nMaximum Scale") -> (0:w51:bool)
      n144 = Greater?(x=w53, y=w54) -> (0:w57:bool)
      n145 = Less?(x=w54, y=w53) -> (x < y?=w52:bool)
      n146 = Select(t="Absolute\nMinimum Score", s=w94, f=w90) -> (s? t:f=w96:dbl)
      "New Min Score" <- w96
      n147 = Or(x=w56, y=w57) -> (x .or. y?=w58:bool)
      n148 = Or(x=w51, y=w52) -> (x .or. y?=w55:bool)
      n149 = Select(t="Absolute\nMinimum Scale", s=w58, f=w53) -> (s? t:f=w74:dbl)
      "New Low Scale" <- w74
      n150 = Select(t="Absolute\nMaximum Scale", s=w55, f=w54) -> (s? t:f=w75:dbl)
      "New high Scale" <- w75
      n151 = Bundle("index"=w92, "Min Scale"=w74, "Max Scale"=w75) -> (w91:T17)  [unwired: 1 in]
      n152 = Replace Array Subset(array=w89, new element=w91, index=w92) -> (w93:T8[])
      n153 = call "IMAQ Overlay ROI"("ROI Descriptor"=w40, "Image"=w73) -> ("Image Out"=→"Right Image 2":T5)  [unwired: 8 in, 1 out]
      n154 = Bundle By Name(cluster="Current Settings", "Range Settings"=w93, "Minimum Match Score"=w96) -> (→"New Settings":T9)
    }
  }
